vi "lab8_task3.vi"() -> ()   [LabVIEW 2021]
uses:
  <vilib>/userDefined/High Color/IMAQdx.ctl
  <vilib>/DAQmx/read.llb/DAQmx Read (Digital Bool 1Line 1Point).vi
  <vilib>/DAQmx/read.llb/DAQmx Read (Analog Wfm 1Chan NSamp).vi
  <vilib>/DAQmx/create/channels.llb/DAQmx Create Channel (AI-Voltage-Basic).vi
  <vilib>/DAQmx/configure/timing.llb/DAQmx Timing (Sample Clock).vi
  <vilib>/DAQmx/configure/trigger.llb/DAQmx Reference Trigger (Digital Edge).vi
  <vilib>/DAQmx/miscellaneous.llb/DAQmx Fill In Error Info.vi
  <vilib>/DAQmx/create/channels.llb/DAQmx Create Channel (DI-Digital Input).vi
  <vilib>/vision/driver/NI_Vision_Acquisition_Software.lvlib
panel:
  in  "Slider":i32(slide)=3 max=199 scale=0.0..199.0
  in  "Stop analysis":bool
  out "Image":T1(plugin-control)
  out "Trigger":bool
  in  "Frames":i32=10
  in  "VideoMode":u32=10
  in  "Session In":T2="cam0"
  in  "rate":dbl=1000.0 format="%0.2f"
  in  "pretrigger samples per channel":u32=500
  out "Waveform Graph":waveform(dbl)(graph)
  in  "# samples to read":i32=1000
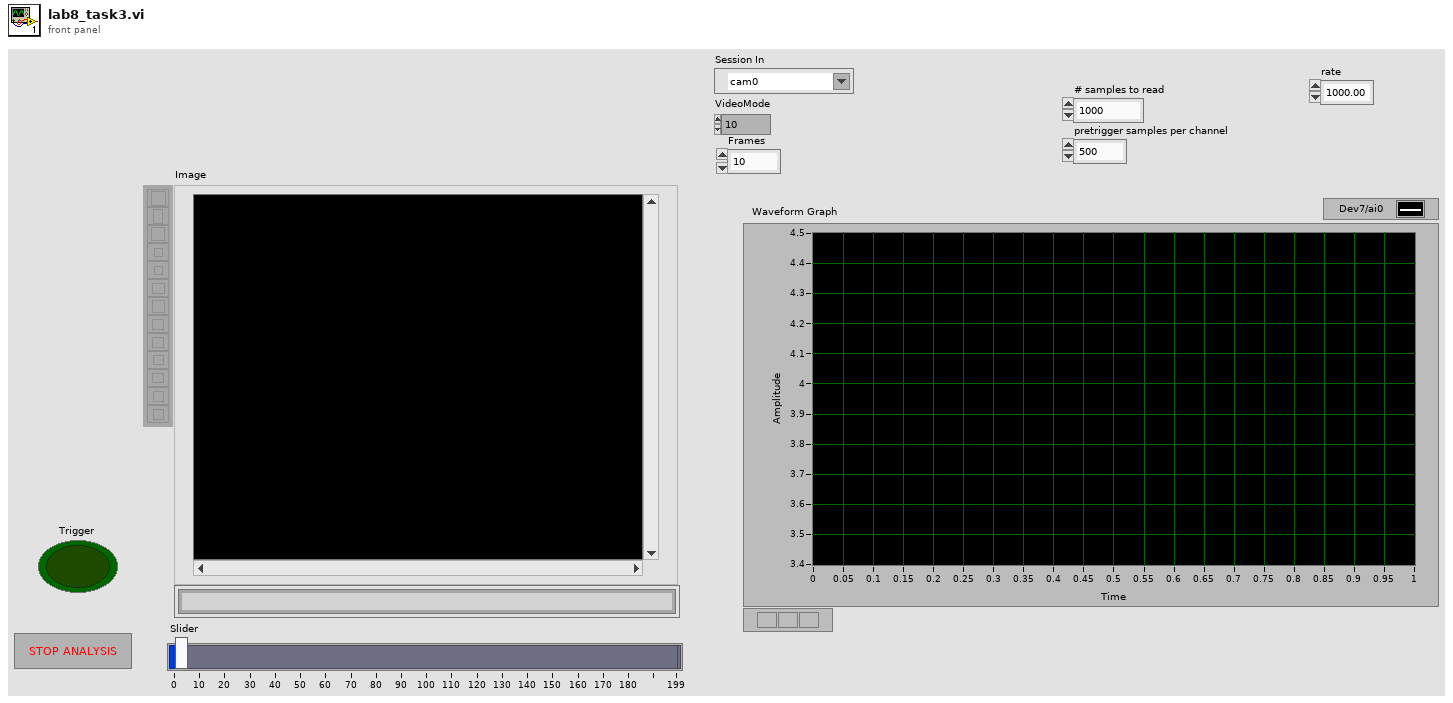
[diagram p1: front panel]
types:
  T1 = typedef "IMAQ Image.ctl" = refnum<image>
  T2 = typedef "IMAQdx.ctl" = refnum<k21>
  T3 = typedef "IMAQ AVI2 Refnum.ctl" = refnum<k20>
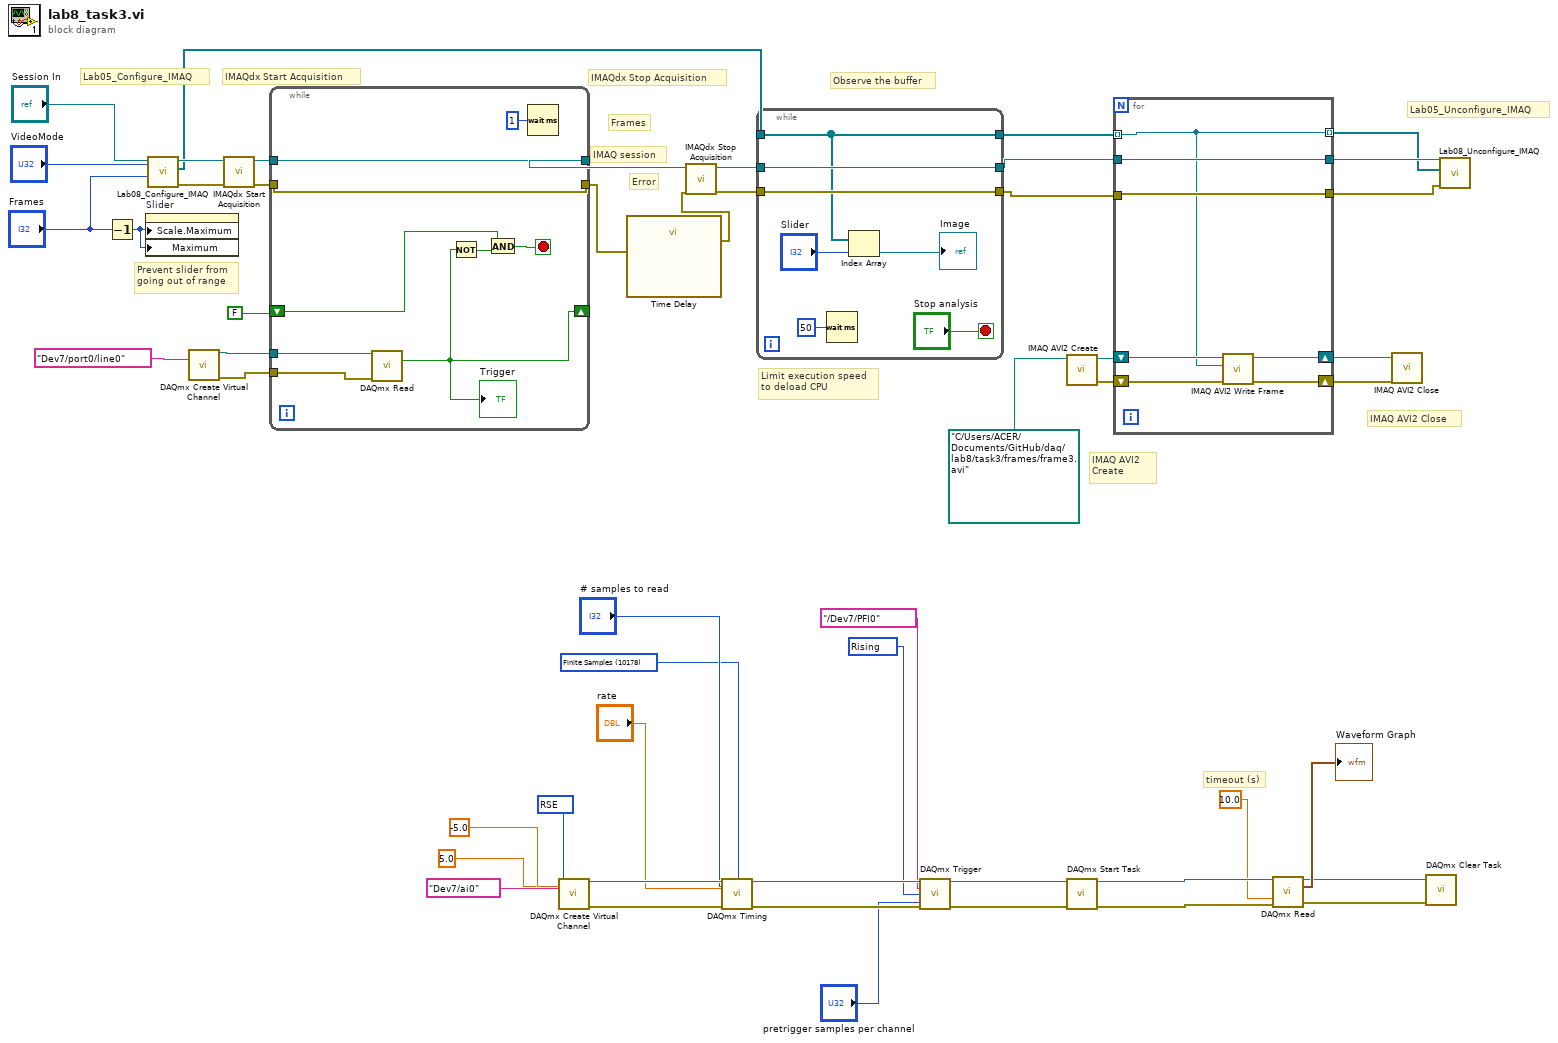
[diagram p0: block diagram]
diagram:
  w42 = 10083 items=["Default"=-1, "RSE"=10083, "NRSE"=10078, "Differential"=10106, "Pseudodifferential"=12529] ("input terminal configuration")
  w43 = 10178 items=["Finite Samples"=10178, "Continuous Samples"=10123, "Hardware Timed Single Point"=12522] ("sample mode")
  w44 = 10280 items=["Rising"=10280, "Falling"=10171] ("edge")
  # "IMAQ AVI2 Create"
  # "IMAQ AVI2 Close"
  # "Limit execution speed\nto deload CPU"
  # "Error"
  # "IMAQ session"
  # "Frames"
  # "Observe the buffer"
  # "Prevent slider from\ngoing out of range"
  # "Lab05_Unconfigure_IMAQ"
  # "Lab05_Configure_IMAQ"
  # "IMAQdx Stop Acquisition"
  # "IMAQdx Start Acquisition"
  # "timeout (s)"
  n1 = Decrement(x="Frames") -> (x-1=w21:i32)
  n2 = property on="Slider" class="Slide (strict)"("Scale.Maximum"=w21, "Maximum"=w21) -> ()  [unwired: 2 in, 2 out]
  n3 = call "Lab08_Configure_IMAQ.vi"("Frames"="Frames", "VideoMode"="VideoMode", "Session In"="Session In") -> ("error out"=w26:errorcluster, "Images Out"=w20:T1[], "Session Out"=w27:T2)  [unwired: 2 in]
  n4 = call-poly <vilib>:"DAQmx Create Virtual Channel.vi"("lines"=tag "Dev7/port0/line0") -> ("task out"=w6:refnum<k21>, "error out"=w5:errorcluster)  [unwired: 13 in]
  n5 = call <vilib>:"IMAQdx Start Acquisition.vi"("error in"=w26, "Session In"=w27) -> ("error out"=w24:errorcluster, "Session Out"=w25:T2)  [unwired: 8 out]
  n6 = while {
    tunnel: w25 -> [w59]
    tunnel: w24 -> [w60]
    tunnel: [w60] -> w2
    tunnel: [w59] -> w23
    tunnel: w6 -> [w57]
    tunnel: w5 -> [w56]
    shift-right: [w53] -> _
    shift-left: FALSE ("data") -> [w52]
    stop <- w55 stop-if-true
    n7 = call-poly <vilib>:"DAQmx Read.vi"("task/channels in"=w57, "error in"=w56) -> ("data"=w53:bool)  [unwired: 11 in, 2 out]
    "Trigger" <- w53
    n8 = Not(x=w53) -> (.not. x?=w54:bool)
    n9 = And(x=w52, y=w54) -> (x .and. y?=w55:bool)
    n10 = Wait (ms)(milliseconds to wait=u32 1) -> ()  [unwired: 1 out]
  }
  n11 = call-poly <vilib>:"DAQmx Create Virtual Channel.vi"("maximum value"=5.0, "minimum value"=-5.0, "input terminal configuration"=w42, "physical channels"=tag "Dev7/ai0") -> ("task out"=w48:refnum<k21>, "error out"=w51:errorcluster)  [unwired: 10 in]
  n12 = call "Time Delay"("error in (no error)"=w2) -> ("error out"=w1:errorcluster)  [unwired: 10 in]
  n13 = call <vilib>:"IMAQdx Stop Acquisition.vi"("error in"=w1, "Session In"=w23) -> ("error out"=w18:errorcluster, "Session Out"=w19:T2)  [unwired: 8 out]
  n14 = call-poly <vilib>:"DAQmx Timing.vi"("task/channels in"=w48, "sample mode"=w43, "samples per channel"="# samples to read", "rate"="rate", "error in"=w51) -> ("task out"=w47:refnum<k21>, "error out"=w50:errorcluster)  [unwired: 9 in]
  n15 = while {
    tunnel: w20 -> [w62]
    tunnel: [w62] -> w10
    tunnel: w19 -> [w64]
    tunnel: [w64] -> w11
    tunnel: w18 -> [w63]
    tunnel: [w63] -> w12
    stop <- "Stop analysis" stop-if-true
    n16 = Wait (ms)(milliseconds to wait=u32 50) -> ()  [unwired: 1 out]
    n17 = Index Array "Index Array"(array=w62, index="Slider") -> (element=→"Image":T1)
  }
  n18 = call-poly <vilib>:"DAQmx Trigger.vi"("task/channels in"=w47, "source"=tag "/Dev7/PFI0", "edge"=w44, "error in"=w50, "pretrigger samples per channel"="pretrigger samples per channel") -> ("task out"=w46:refnum<k21>, "error out"=w49:errorcluster)  [unwired: 9 in]
  n19 = call "IMAQ AVI2 Create"("AVI Path"=path "C:/Users/ACER/Documents/GitHub/daq/lab8/task3/frames/frame3.avi") -> ("error out"=w15:errorcluster, "AVI Refnum"=w14:T3)  [unwired: 9 in]
  n20 = call <vilib>:"DAQmx Start Task.vi"("task/channels in"=w46, "error in"=w49) -> ("task out"=w36:refnum<k21>, "error out"=w37:errorcluster)  [unwired: 12 in]
  n21 = for {
    shift-right: [w74] -> w17
    shift-left: w14 -> [w71]
    shift-right: [w73] -> w16
    shift-left: w15 -> [w72]
    tunnel: w12 -> [w70]
    tunnel: w11 -> [w69]
    tunnel: w10 -> [w68] mode=indexing
    tunnel: [w70] -> w9
    tunnel: [w69] -> w8
    tunnel: [w68] -> w7 mode=indexing
    n22 = call "IMAQ AVI2 Write Frame"("error in (no error)"=w72, "Image"=w68, "AVI Refnum"=w71) -> ("error out"=w73:errorcluster, "AVI Refnum (duplicate)"=w74:T3)  [unwired: 6 in, 1 out]
  }
  n23 = call-poly <vilib>:"DAQmx Read.vi"("task/channels in"=w36, "timeout"=10.0, "error in"=w37) -> ("task out"=w33:refnum<k21>, "data"=→"Waveform Graph":waveform(dbl), "error out"=w32:errorcluster)  [unwired: 10 in]
  n24 = call "IMAQ AVI2 Close"("error in (no error)"=w16, "AVI Refnum"=w17) -> ()  [unwired: 9 in, 1 out]
  n25 = call <vilib>:"DAQmx Clear Task.vi"("task in"=w33, "error in"=w32) -> ()  [unwired: 13 in, 1 out]
  n26 = call "Lab08_Unconfigure_IMAQ.vi"("error in (no error)"=w9, "Images to dispose"=w7, "IMAQdx session in"=w8) -> ()  [unwired: 8 in, 1 out]
